vi "test Acyclic Loopback.vi"(8 "error in":errorcluster, 11 "TestCase in":refnum<class "Single Board 1Ch Loopback.lvclass">) -> (0 "error out":errorcluster, 3 "TestCase out":refnum<class "Single Board 1Ch Loopback.lvclass">)   [LabVIEW 2020, in "Single Board 1Ch Loopback.lvclass"]
uses:
  Single Board 1Ch Loopback.lvclass
  C:/dev/git/niveristand-custom-device-testing-tools/VeriStandTestCase/VeriStandTestCase.lvclass
  <vilib>/numeric/Random Number (Range) U64.vi
  <vilib>/numeric/sub_Random U32.vi
  <vilib>/NI VeriStand/Execution/Workspace/NI VeriStand - Set Multiple Channel Values.vi
  <vilib>/addons/_JKI Toolkits/VI Tester/TestCase.llb/TestCase.lvclass
  <vilib>/NI VeriStand/Execution/Workspace/NI_VS Workspace ExecutionAPI.lvlib
  niveristand-custom-device-testing-tools/VeriStandTestUtilities/VeriStandTestUtilities.lvlib
  C:/Program Files (x86)/National Instruments/LabVIEW 2020/vi.lib/addons/_JKI Toolkits/VI Tester/TestCase.llb/TestCase.lvclass
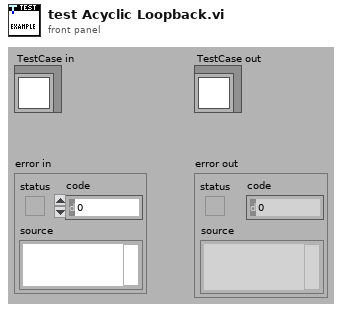
[diagram p1: front panel]
types:
  T1 = typedef "NI_VS Workspace ExecutionAPI.lvlib/WorkspaceAPI.ctl" = refnum<k24>
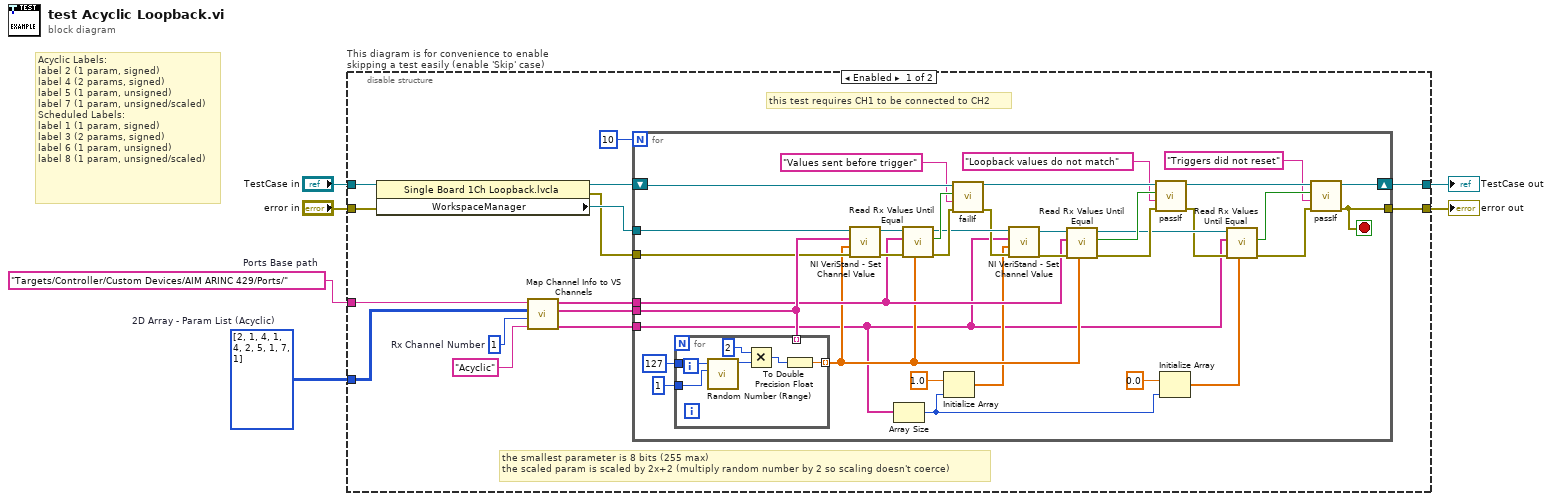
[diagram p0: block diagram]
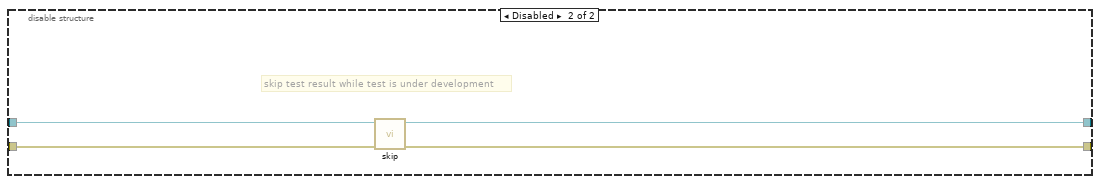
[diagram p2: hidden frame]
diagram:
  w2 = i32[][] [[2, 1], [4, 1], [4, 2], [5, 1], [7, 1]]  # 2D Array - Param List (Acyclic)
  w3 = "Targets/Controller/Custom Devices/AIM ARINC 429/Ports/"  # Ports Base path
  # "Acyclic Labels:\nlabel 2 (1 param, signed)\nlabel 4 (2 params, signed)\nlabel 5 (1 param, unsigned)\nlabel 7 (1 param, unsigned/scaled)\nScheduled Labels:\nlabel 1 (1 param, signed)\nlabel 3 (2 params, signed)\nlabel 6 (1 param, unsigned)\nlabel 8 (1 param, unsigned/scaled)"
  n1 = disable-structure "This diagram is for convenience to enable skipping a test easily (enable 'Skip' case)" shown="Enabled" {
    disable-tunnel: "TestCase in" -> [w15 w66]
    disable-tunnel: [w13 w64] -> w1
    disable-tunnel: [w12 w65] -> w5
    disable-tunnel: "error in" -> [w14 w63]
    disable-tunnel: w3 -> [w16 _]
    disable-tunnel: w2 -> [w9 _]
    frame Enabled {
      w10 = 1  # Rx Channel Number
      # "this test requires CH1 to be connected to CH2"
      # "the smallest parameter is 8 bits (255 max)\nthe scaled param is scaled by 2x+2 (multiply random number by 2 so scaling doesn't coerce)"
      n2 = property class="Single Board 1Ch Loopback.lvcla"(reference=w15, error in=w14) -> (reference out=w18:refnum<class "Single Board 1Ch Loopback.lvclass">, error out=w19:errorcluster, "WorkspaceManager"=w20:T1)
      n3 = call "Map Channel Info to VS Channels.vi"("Transfer Type"="Acyclic", "Rx Channel Number"=w10, "2D Array - Label/Param List"=w9, "VS Channel Base Port"=w16) -> ("Tx Trigger Channels Array"=w7:string[], "Tx Channels Array"=w8:string[], "Rx Channels Array"=w21:string[])  [unwired: 4 in, 1 out]
      n4 = for {
        N: 10 -> [_]
        tunnel: w21 -> [w42]
        tunnel: w20 -> [w54]
        tunnel: w19 -> [w47]
        tunnel: w8 -> [w53]
        shift-right: [w35] -> w13
        shift-left: w18 -> [w49]
        tunnel: [w37] -> w12
        tunnel: w7 -> [w25]
        stop <- w37 stop-if-true
        n5 = for {
          tunnel: [w61] -> w41 mode=indexing
          tunnel: u64 127 ("upper bound (100)") -> [w60]
          tunnel: u64 1 ("upper bound (100)") -> [w59]
          tunnel: w53 -> [_] mode=indexing
          n6 = call-poly <vilib>:"Random Number (Range).vi"("lower bound (0)"=w59, "upper bound (100)"=w60) -> ("number"=w62:u64)  [unwired: 9 in]
          n7 = Multiply(x=u64 2, y=w62) -> (x*y=w58:u64)
          n8 = To Double Precision Float(number=w58) -> (double precision float=w61:dbl)
        }
        n9 = call-poly <vilib>:"NI VeriStand - Set Channel Value.vi"("error in (no error)"=w47, "Values"=w41, "Channels"=w53, "WorkspaceManager in"=w54) -> ("error out"=w50:errorcluster, "WorkspaceManager out"=w52:T1)  [unwired: 6 in]
        n10 = Array Size(array=w25) -> (size(s)=w22:i32)
        n11 = call "Read Rx Values Until Equal.vi"("expected values"=w41, "error in"=w50, "Rx aliases"=w42, "workspace manager in"=w52) -> ("error out"=w51:errorcluster, "values equal expected"=w48:bool, "workspace manager out"=w46:T1)  [unwired: 5 in]
        n12 = Initialize Array(1.0, w22) -> (w26:dbl[])
        n13 = call-dynamic "failIf.vi"("error in (no error)"=w51, "message (\"\")"="Values sent before trigger" ("message (\"\")"), "fail"=w48, "TestCase in"=w49) -> ("error out"=w45:errorcluster, "TestCase out"=w38:refnum<class "Single Board 1Ch Loopback.lvclass">)  [unwired: 6 in]
        n14 = call-poly <vilib>:"NI VeriStand - Set Channel Value.vi"("error in (no error)"=w45, "Values"=w26, "Channels"=w25, "WorkspaceManager in"=w46) -> ("error out"=w43:errorcluster, "WorkspaceManager out"=w44:T1)  [unwired: 6 in]
        n15 = call "Read Rx Values Until Equal.vi"("expected values"=w41, "error in"=w43, "Rx aliases"=w42, "workspace manager in"=w44) -> ("error out"=w39:errorcluster, "values equal expected"=w40:bool, "workspace manager out"=w33:T1)  [unwired: 5 in]
        n16 = call-dynamic "passIf.vi"("error in (no error)"=w39, "message (\"\")"="Loopback values do not match" ("message (\"\")"), "pass"=w40, "TestCase in"=w38) -> ("error out"=w32:errorcluster, "TestCase out"=w36:refnum<class "Single Board 1Ch Loopback.lvclass">)  [unwired: 6 in]
        n17 = Initialize Array(0.0, w22) -> (w23:dbl[])
        n18 = call "Read Rx Values Until Equal.vi"("expected values"=w23, "error in"=w32, "Rx aliases"=w25, "workspace manager in"=w33) -> ("error out"=w31:errorcluster, "values equal expected"=w34:bool)  [unwired: 5 in, 1 out]
        n19 = call-dynamic "passIf.vi"("error in (no error)"=w31, "message (\"\")"="Triggers did not reset" ("message (\"\")"), "pass"=w34, "TestCase in"=w36) -> ("error out"=w37:errorcluster, "TestCase out"=w35:refnum<class "Single Board 1Ch Loopback.lvclass">)  [unwired: 6 in]
      }
    }
    frame Disabled {
      # "skip test result while test is under development"
      n20 = call <vilib>:"skip.vi"("error in (no error)"=w63, "TestCase in"=w66) -> ("error out"=w65:errorcluster, "TestCase out"=w64:refnum<class "Single Board 1Ch Loopback.lvclass">)  [unwired: 8 in]
    }
  }
  "error out" <- w5
  "TestCase out" <- w1
